vi "PTScanner.ProcDestructor.vi"(0 "i ref in":refnum<vi>, 5 "error in (no error)":errorcluster) -> (14 "i ref out":refnum<vi>, 19 "error out":errorcluster)   [LabVIEW 2014, in "PTScanner.lvlib"]
uses:
  PTScanner.lvlib
  PTScanner.obj parameters.ctl
  CSlibraries-extern/DimLVEvent/LVDimInterface/LVDimInterface.lvlib
  CS_Core/BaseSM/BaseSM.lvlib
panel:
  in  "Objects":T1[](array[typedef])
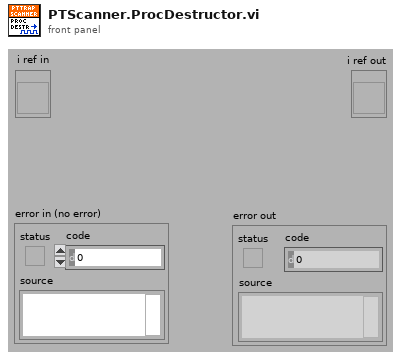
[diagram p1: front panel]
types:
  T1 = typedef "PTScanner.lvlib/PTScanner.obj parameters.ctl" = cluster{"object":string, "DIM address":string, "method":string, "data descriptor":string, "method parameters":cluster{"Name":string, "Descr":string, "Value":string, "Value?":bool}[], "Call Mode":enum16{"Simple DIM", "Synchronous"}, "actValue":dbl, "Centroid":dbl, "Minus Delta":dbl, "Plus Delta":dbl, "increment":dbl, "DIM Status":cluster{"no link":bool, "quality":i32, "Time Stamp":timestamp}, "range":dbl, "DIMChannelIndex":i32}
  T2 = typedef "PTScanner.lvlib/PTScanner.i attribute.ctl" = cluster{"Object cmds":T1[], "Steps":cluster{"Finished":bool, "cmd setup":T3[]}[], "curStep":i32, "DIM IDs":cluster{"AllFinished":i32, "Finished":i32, "curStep":i32, "nofSteps":i32, "NomValues":i32[], "1D-Min":i32, "1D-Max":i32, "Dimensions":i32, "MaxDimensions":i32, "ScanedDeviceNames":i32[]}, "All Finished":bool, "DIMs in use":string[], "Running":bool, "Scan Delay":u32, "loop":bool, "Paused":bool, "Formed":bool}
  T3 = typedef "PTScanner.lvlib/PTScanner.step obj parameters.ctl" = cluster{"obj index":i32, "nomValue":dbl, "fulfilled":bool}
  T4 = cluster{"AllFinished":i32, "Finished":i32, "curStep":i32, "nofSteps":i32, "NomValues":i32[], "1D-Min":i32, "1D-Max":i32, "Dimensions":i32, "MaxDimensions":i32, "ScanedDeviceNames":i32[]}
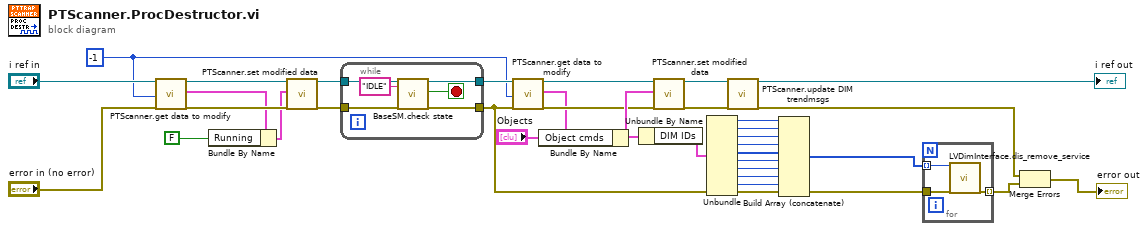
[diagram p0: block diagram]
diagram:
  w13 = -1 ("ms timeout (10000)")
  n1 = call "PTScanner.get data to modify.vi"("i ref in"="i ref in", "ms timeout (10000)"=w13, "error in (no error)"="error in (no error)") -> ("i ref out"=w32:refnum<vi>, "i attribute"=w29:T2, "error out"=w31:errorcluster)  [unwired: 13 in, 1 out]
  n2 = Bundle By Name(cluster=w29, "Running"=FALSE) -> (w30:T2)
  n3 = call "PTScanner.set modified data.vi"("i ref in"=w32, "CLASS.i attribute"=w30, "error in (no error)"=w31) -> ("i ref out"=w26:refnum<vi>, "error out"=w25:errorcluster)  [unwired: 15 in]
  n4 = while {
    tunnel: w26 -> [w39]
    tunnel: w25 -> [w38]
    tunnel: [w37] -> w15
    tunnel: [w36] -> w14
    stop <- w41 stop-if-true
    n5 = call "BaseSM.check state.vi"("i ref in"=w39, "requestedState"="IDLE", "error in (no error)"=w38) -> ("i ref out"=w36:refnum<vi>, "OK"=w41:bool, "error out"=w37:errorcluster)  [unwired: 11 in, 3 out]
  }
  n6 = call "PTScanner.get data to modify.vi"("i ref in"=w14, "ms timeout (10000)"=w13, "error in (no error)"=w15) -> ("i ref out"=w24:refnum<vi>, "i attribute"=w20:T2, "error out"=w21:errorcluster)  [unwired: 13 in, 1 out]
  n7 = Bundle By Name(cluster=w20, "Object cmds"="Objects") -> (w22:T2)
  n8 = Unbundle By Name(w20) -> ("DIM IDs"=w12:T4)
  n9 = call "PTScanner.set modified data.vi"("i ref in"=w24, "CLASS.i attribute"=w22, "error in (no error)"=w21) -> ("i ref out"=w19:refnum<vi>, "error out"=w16:errorcluster)  [unwired: 15 in]
  n10 = Unbundle(w12) -> ("AllFinished"=w11:i32, "Finished"=w10:i32, "curStep"=w9:i32, "nofSteps"=w8:i32, "NomValues"=w7:i32[], "1D-Min"=w5:i32, "1D-Max"=w4:i32, "Dimensions"=w3:i32, "MaxDimensions"=w2:i32, "ScanedDeviceNames"=w1:i32[])
  n11 = call "PTScanner.update DIM trendmsgs.vi"("i ref in"=w19, "error in"=w16) -> ("i ref out"=→"i ref out":refnum<vi>, "error out"=w17:errorcluster)  [unwired: 16 in]
  n12 = Build Array (concatenate)(w11, w10, w9, w8, w7, w5, w4, w3, w2, w1) -> (w6:i32[])
  n13 = for {
    tunnel: w6 -> [w44] mode=indexing
    tunnel: [w43] -> w35 mode=indexing
    tunnel: w15 -> [w42]
    n14 = call "LVDimInterface.dis_remove_service.vi"("my_serviceID"=w44, "error in (no error)"=w42) -> ("error out"=w43:errorcluster)  [unwired: 17 in]
  }
  n15 = Merge Errors(w17, w35) -> (→"error out":errorcluster)
